vi "Read N.vi"(8 "error in (no error)":errorcluster, 11 "Online_SNR in":refnum<class "Online_SNR.lvclass">) -> (0 "error out":errorcluster, 2 "N":dbl, 3 "Online_SNR out":refnum<class "Online_SNR.lvclass">)   [LabVIEW 2021, in "Online_SNR.lvclass"]
uses:
  Online_SNR.lvclass
  Online_SNR.lvclass/Online_SNR.ctl
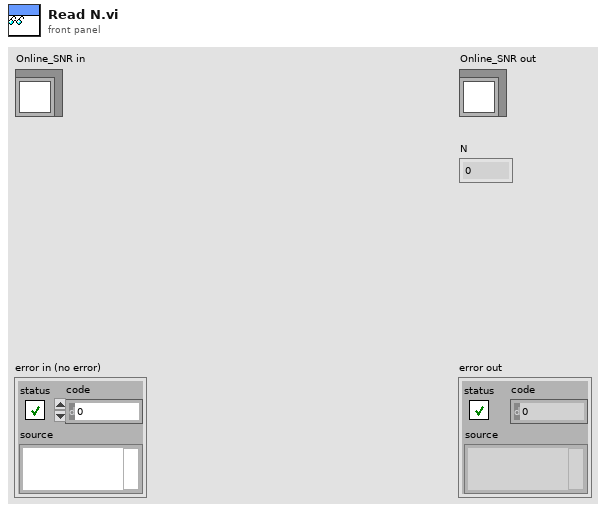
[diagram p1: front panel]
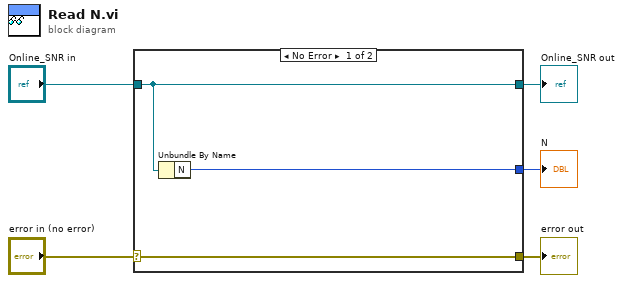
[diagram p0: block diagram]
diagram:
  n1 = case shown="No Error" "error in (no error)" {
    selector: "error in (no error)" -> [w8 w9]
    tunnel: [w8 w9] -> w4
    tunnel: [w7 w10] -> w2
    tunnel: "Online_SNR in" -> [w7 w10]
    tunnel: [w6 _] -> w1
    frame No Error {
      n2 = Unbundle By Name(w7) -> ("N"=w6:i64)
    }
    frame Error {
    }
  }
  "error out" <- w4
  "Online_SNR out" <- w2
  "N" <- w1
